vi "Move Axis_G.vi"(8 "error in (no error)":errorcluster, 9 "Where, mm":dbl, 10 "Axis":i32, 11 "Control-Client in":refnum<class "Control-Client.lvclass">) -> (0 "error out":errorcluster, 3 "Control-Client out":refnum<class "Control-Client.lvclass">)   [LabVIEW 2019, in "Control-Client.lvclass"]
uses:
  Control-Client.lvclass
  dependecies/ControlsVIs/Clusters-def/Message types.ctl
  dependecies/ControlsVIs/Clusters-def/SERVER-Commands.ctl
  dependecies/ControlsVIs/Clusters-def/DL-Com-MoveAxis.ctl
  Control-Server/Control-Server.lvclass
  Delay Line/DelayLine.lvclass
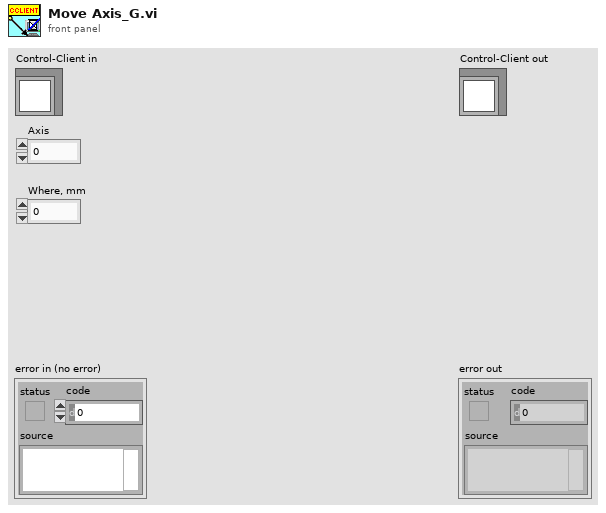
[diagram p1: front panel]
types:
  T1 = typedef "DelayLine.lvclass/DL-Com-MoveAxis.ctl" = cluster{"Axis":i32, "Where":dbl, "How":u16}
  T2 = typedef "Control-Server.lvclass/SERVER-Commands.ctl" = string
  T3 = typedef "Message types.ctl" = string
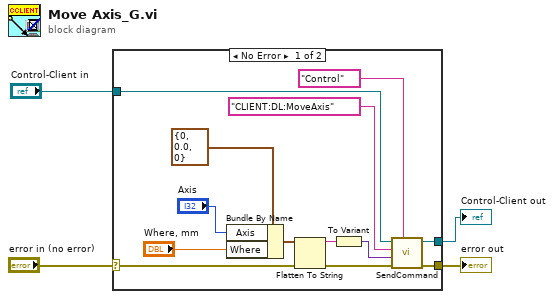
[diagram p0: block diagram]
diagram:
  n1 = case shown="No Error" "error in (no error)" {
    selector: "error in (no error)" -> [w6 w19]
    tunnel: [w11 w19] -> w3
    tunnel: [w9 w18] -> w1
    tunnel: "Control-Client in" -> [w10 w18]
    frame No Error {
      n2 = Bundle By Name(cluster=T1 {"Axis"=0, "Where"=0.0, "How"=0} ("output cluster"), "Axis"="Axis", "Where"="Where, mm") -> (w13:T1)
      n3 = Flatten To String(anything=w13, error in (no error)=w6) -> (data string=w12:string, error out=w5:errorcluster)  [unwired: 2 in, 1 out]
      n4 = To Variant(anything=w12) -> (Variant=w14:variant)
      n5 = call "SendCommand.vi"("Message type"=T3 "Control", "error in (no error)"=w5, "data"=w14, "Command"=T2 "CLIENT:DL:MoveAxis" ("Commands"), "Control-Client in"=w10) -> ("error out"=w11:errorcluster, "Control-Client out"=w9:refnum<class "Control-Client.lvclass">)  [unwired: 5 in]
    }
    frame Error {
    }
  }
  "error out" <- w3
  "Control-Client out" <- w1
